vi "CreateFileName.vi"(8 "error in (no error)":errorcluster, 10 "Date":string, 11 "Interface.lvclass":refnum<class "Interface.lvclass">) -> (0 "error out":errorcluster, 3 "Interface.lvclass Out":refnum<class "Interface.lvclass">)   [LabVIEW 2010, in "Interface.lvclass"]
doc: "Ce VI sauvegarde les données d'acquisition pour en garder une copie de sécurité qui peut être rappeller en cas de panne."
uses:
  Interface.lvclass
  Interface.lvclass/Interface.ctl
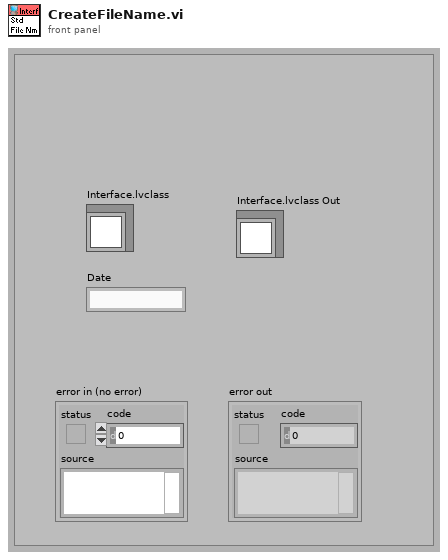
[diagram p1: front panel]
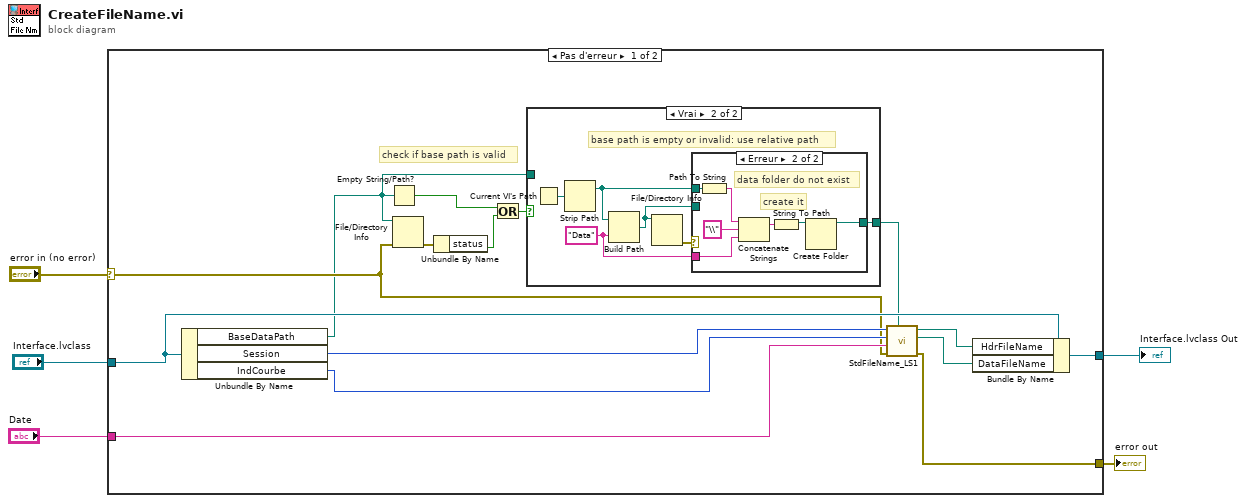
[diagram p0: block diagram]
diagram:
  n1 = case shown="Pas d'erreur" "error in (no error)" {
    selector: "error in (no error)" -> [w7 w37]
    tunnel: [w12 w37] -> w4
    tunnel: "Date" -> [w9 _]
    tunnel: "Interface.lvclass" -> [w16 w36]
    tunnel: [w15 w36] -> w1
    frame No Error {
      # "check if base path is valid"
      n2 = Unbundle By Name(w16) -> ("BaseDataPath"=w6:path, "Session"=w14:i32, "IndCourbe"=w13:i64)
      n3 = Empty String/Path?(string/path=w6) -> (empty?=w20:bool)
      n4 = File/Directory Info(path=w6, error in=w7) -> (error out=w19:errorcluster)  [unwired: 6 out]
      n5 = Unbundle By Name(w19) -> ("status"=w18:bool)
      n6 = Or(x=w20, y=w18) -> (x .or. y?=w17:bool)
      n7 = case shown="Vrai" w17 {
        tunnel: [w21 w26] -> w8
        tunnel: w6 -> [w21 _]
        frame False {
          # "basepath valid: use it"
        }
        frame True {
          w24 = "Data" ("nom ou chemin relatif")
          # "base path is empty or invalid: use relative path"
          n8 = Current VI's Path() -> (path=w27:path)
          n9 = Strip Path(path=w27) -> (stripped path=w25:path)  [unwired: 1 out]
          n10 = Build Path(base path=w25, name or relative path=w24) -> (appended path=w22:path)
          n11 = File/Directory Info(path=w22) -> (error out=w23:errorcluster)  [unwired: 1 in, 6 out]
          n12 = case shown="Erreur" w23 {
            tunnel: [w28 w35] -> w26
            tunnel: w25 -> [_ w34]
            tunnel: w24 -> [_ w30]
            tunnel: w22 -> [w28 _]
            frame No Error {
            }
            frame Error {
              # "create it"
              # "data folder do not exist"
              n13 = Path To String(path=w34) -> (string=w33:string)
              n14 = Concatenate Strings(w33, "\\" ("chaîne"), w30) -> (w32:string)
              n15 = String To Path(string=w32) -> (path=w31:path)
              n16 = Create Folder(path (use dialog)=w31) -> (created path=w35:path)  [unwired: 2 in, 2 out]
            }
          }
        }
      }
      n17 = call "StdFileName_LS1.vi"("chemin de base"=w8, "error in (no error)"=w7, "Date"=w9, "Scan"=w13, "Session"=w14) -> ("error out"=w12:errorcluster, "chemin Data"=w10:path, "chemin Headers"=w11:path)  [unwired: 2 in, 2 out]
      n18 = Bundle By Name(cluster=w16, "HdrFileName"=w11, "DataFileName"=w10) -> (w15:refnum<class "Interface.lvclass">)
    }
    frame Error {
    }
  }
  "error out" <- w4
  "Interface.lvclass Out" <- w1
